vi "button_subvi.vi"() -> ()   [LabVIEW 2023]
panel:
  in  "Stop Button":bool
  # "This is the subvi called\nby button_main.vi"
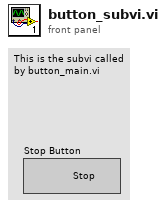
[diagram p1: front panel]
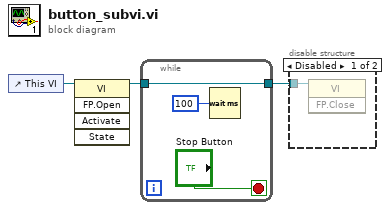
[diagram p0: block diagram]
diagram:
  n1 = control-ref of="This VI"() -> (w3:refnum<vi>)
  n2 = invoke class="VI" method="FP.Open"(reference=w3) -> (reference out=w2:refnum<vi>)  [unwired: 4 in, 4 out]
  n3 = while {
    tunnel: w2 -> [w4]
    tunnel: [w4] -> w1
    stop <- "Stop Button" stop-if-true
    n4 = Wait (ms)(milliseconds to wait=u32 100) -> ()  [unwired: 1 out]
  }
  n5 = disable-structure shown="Disabled" {
    disable-tunnel: w1 -> [w7 _]
    frame Disabled {
      n6 = invoke class="VI" method="FP.Close"(reference=w7) -> ()  [unwired: 2 in, 3 out]
    }
    frame Enabled {
    }
  }
